vi "err_test.vi"() -> ()   [LabVIEW 2020]
panel:
  out "appended array":bool[](array[boolean])
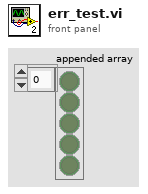
[diagram p1: front panel]
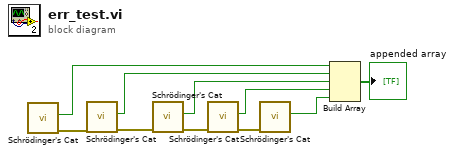
[diagram p0: block diagram]
diagram:
  n1 = call "Schrödinger's Cat.vi"() -> ("error out"=w9:errorcluster, "Boolean"=w6:bool)  [unwired: 10 in]
  n2 = call "Schrödinger's Cat.vi"("error in (no error)"=w9) -> ("error out"=w10:errorcluster, "Boolean"=w5:bool)  [unwired: 9 in]
  n3 = call "Schrödinger's Cat.vi"("error in (no error)"=w10) -> ("error out"=w8:errorcluster, "Boolean"=w4:bool)  [unwired: 9 in]
  n4 = call "Schrödinger's Cat.vi"("error in (no error)"=w8) -> ("error out"=w7:errorcluster, "Boolean"=w3:bool)  [unwired: 9 in]
  n5 = call "Schrödinger's Cat.vi"("error in (no error)"=w7) -> ("Boolean"=w2:bool)  [unwired: 9 in, 1 out]
  n6 = Build Array(w6, w5, w4, w3, w2) -> (→"appended array":bool[])
